vi "TrajectoryParam_calcStuffRev.vi"(6 "TRAJECTORY_CONFIG":T1 {"End Velocity" format="%20.4f"; "StartVelocity" format="%20.4f"; "Max Acceleration" format="%20.4f"; "MaxVelocity" format="%20.4f"}, 7 "Reversed":bool, 9 "successorCONSTRAINED_STATEin":T2={"POSEwCURVATURE"={"CURVATURE"=0.0, "POSE"={"TRANSLATION"={"X"=0.0, "Y"=0.0}, "ROTATION"={"VALUE"=0.0, "COS"=1.0, "SIN"=0.0}}}, "Distance"=0.0, "minAccel"=0.0, "maxAccel"=0.0, "maxVelocity"=0.0} {"POSEwCURVATURE"."POSE"."ROTATION"."SIN" format="%13.4f"; "POSEwCURVATURE"."POSE"."ROTATION"."COS" format="%13.4f"; "POSEwCURVATURE"."POSE"."ROTATION"."VALUE" format="%13.4f"; "POSEwCURVATURE"."POSE"."TRANSLATION"."Y" format="%14.3f"; "POSEwCURVATURE"."POSE"."TRANSLATION"."X" format="%14.3f"}, 11 "thisCONSTRAINED_STATEin":T2={"POSEwCURVATURE"={"CURVATURE"=0.0, "POSE"={"TRANSLATION"={"X"=0.0, "Y"=0.0}, "ROTATION"={"VALUE"=0.0, "COS"=1.0, "SIN"=0.0}}}, "Distance"=0.0, "minAccel"=0.0, "maxAccel"=0.0, "maxVelocity"=0.0} {"POSEwCURVATURE"."POSE"."ROTATION"."SIN" format="%13.4f"; "POSEwCURVATURE"."POSE"."ROTATION"."COS" format="%13.4f"; "POSEwCURVATURE"."POSE"."ROTATION"."VALUE" format="%13.4f"; "POSEwCURVATURE"."POSE"."TRANSLATION"."Y" format="%14.3f"; "POSEwCURVATURE"."POSE"."TRANSLATION"."X" format="%14.3f"}) -> (0 "error out":errorcluster, 1 "successorCONSTRAINED_STATEout":T2={"POSEwCURVATURE"={"CURVATURE"=0.0, "POSE"={"TRANSLATION"={"X"=0.0, "Y"=0.0}, "ROTATION"={"VALUE"=0.0, "COS"=1.0, "SIN"=0.0}}}, "Distance"=0.0, "minAccel"=0.0, "maxAccel"=0.0, "maxVelocity"=0.0} {"POSEwCURVATURE"."POSE"."ROTATION"."SIN" format="%13.4f"; "POSEwCURVATURE"."POSE"."ROTATION"."COS" format="%13.4f"; "POSEwCURVATURE"."POSE"."ROTATION"."VALUE" format="%13.4f"; "POSEwCURVATURE"."POSE"."TRANSLATION"."Y" format="%14.3f"; "POSEwCURVATURE"."POSE"."TRANSLATION"."X" format="%14.3f"}, 3 "thisCONSTRAINED_STATEout":T2={"POSEwCURVATURE"={"CURVATURE"=0.0, "POSE"={"TRANSLATION"={"X"=0.0, "Y"=0.0}, "ROTATION"={"VALUE"=0.0, "COS"=1.0, "SIN"=0.0}}}, "Distance"=0.0, "minAccel"=0.0, "maxAccel"=0.0, "maxVelocity"=0.0} {"POSEwCURVATURE"."POSE"."ROTATION"."SIN" format="%13.4f"; "POSEwCURVATURE"."POSE"."ROTATION"."COS" format="%13.4f"; "POSEwCURVATURE"."POSE"."ROTATION"."VALUE" format="%13.4f"; "POSEwCURVATURE"."POSE"."TRANSLATION"."Y" format="%14.3f"; "POSEwCURVATURE"."POSE"."TRANSLATION"."X" format="%14.3f"})   [LabVIEW 2019, in "Trajectory_Library.lvlib"]
doc: "Internal routine called by TrajectoryParam_timeParam.VI"
uses:
  Trajectory_Library.lvlib
  CONSTRAINED_STATE.ctl
  POSEwCURVATURE.ctl
  POSE2D.ctl
  TRANSLATION2D.ctl
  ROTATION2D.ctl
  TRAJ_CONFIG.ctl
panel:
  # "All units\nare SI"
  # "All units\nare SI"
  # "All units\nare SI"
  # "All units\nare SI"
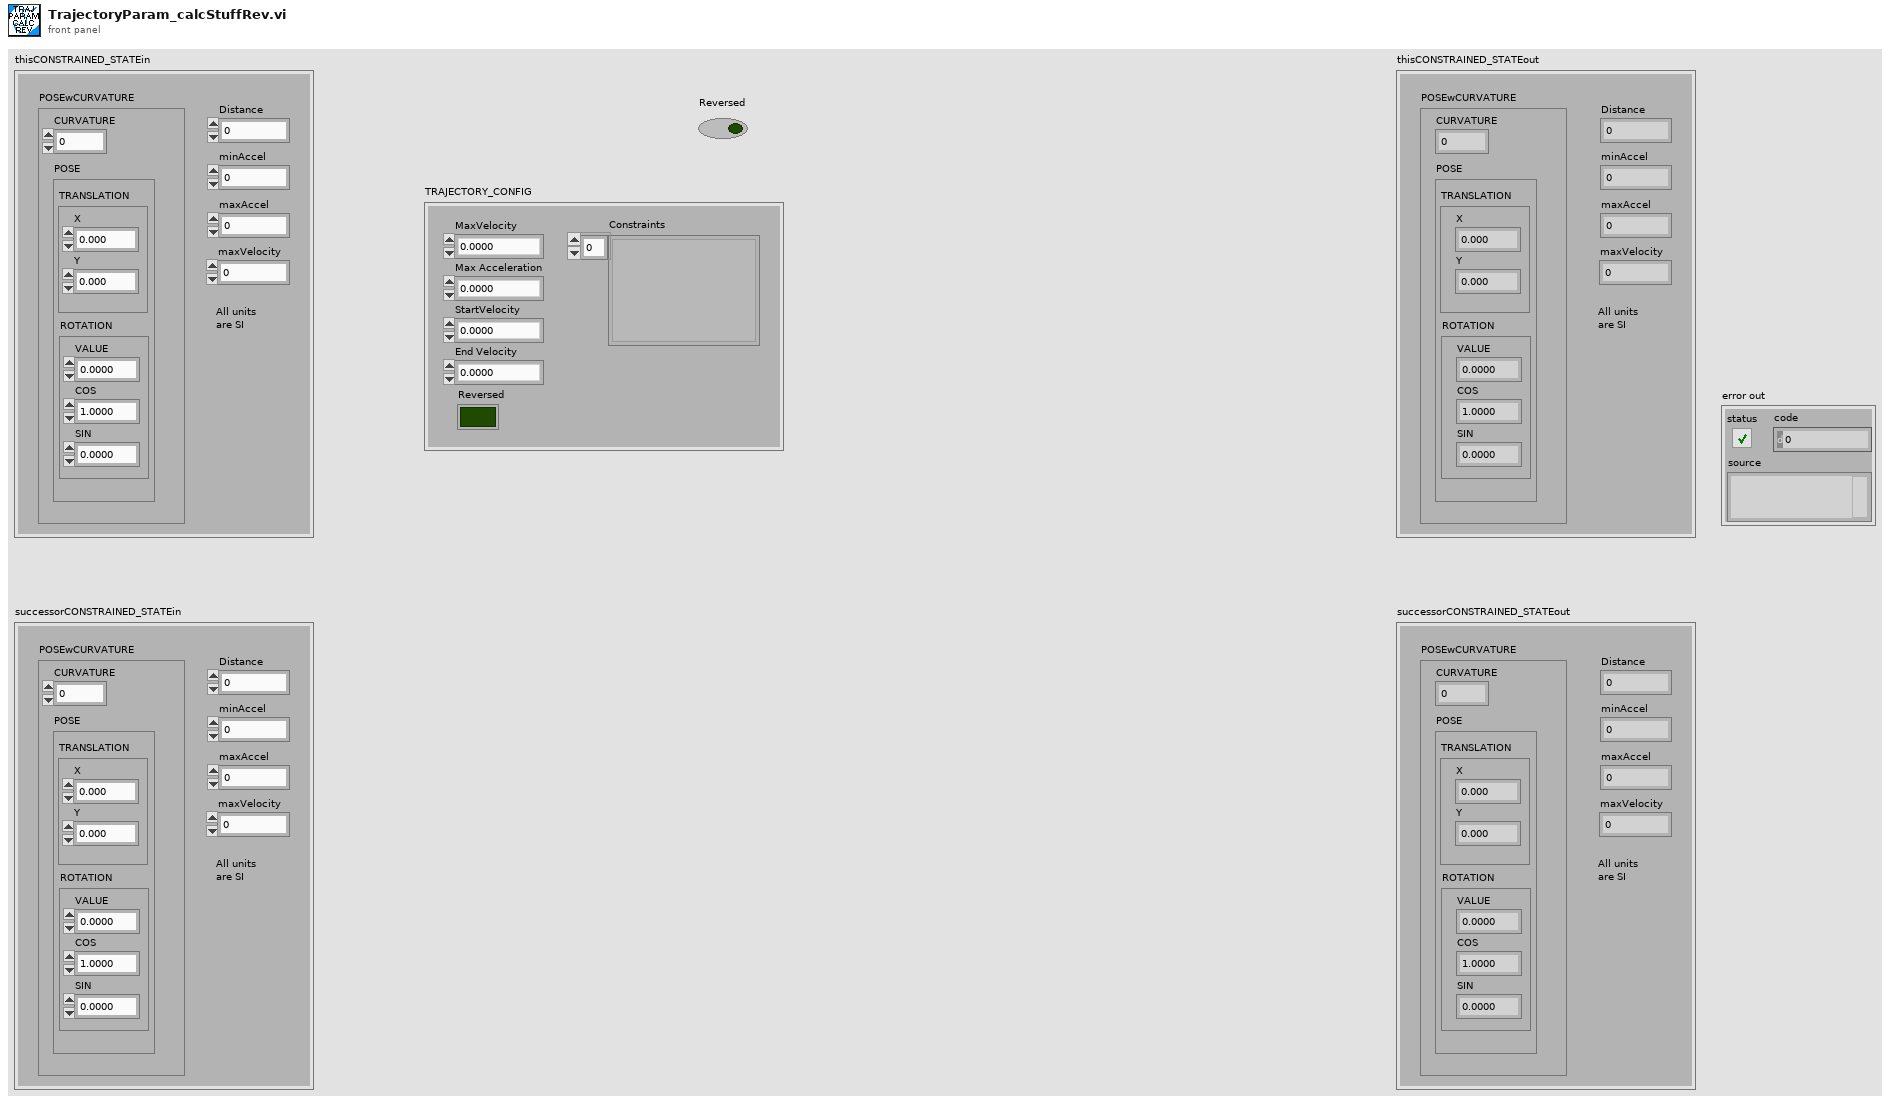
[diagram p1: front panel]
types:
  T1 = typedef "Trajectory_Library.lvlib/TRAJ_CONFIG.ctl" = cluster{"MaxVelocity":dbl, "Max Acceleration":dbl, "StartVelocity":dbl, "End Velocity":dbl, "Reversed":bool, "Constraints":variant[]}
  T2 = typedef "Trajectory_Library.lvlib/CONSTRAINED_STATE.ctl" = cluster{"POSEwCURVATURE":T3, "Distance":dbl, "minAccel":dbl, "maxAccel":dbl, "maxVelocity":dbl}
  T3 = typedef "Trajectory_Library.lvlib/POSEwCURVATURE.ctl" = cluster{"CURVATURE":dbl, "POSE":T4}
  T4 = typedef "Trajectory_Library.lvlib/POSE2D.ctl" = cluster{"TRANSLATION":T5, "ROTATION":T6}
  T5 = typedef "Trajectory_Library.lvlib/TRANSLATION2D.ctl" = cluster{"X":dbl, "Y":dbl}
  T6 = typedef "Trajectory_Library.lvlib/ROTATION2D.ctl" = cluster{"VALUE":dbl, "COS":dbl, "SIN":dbl}
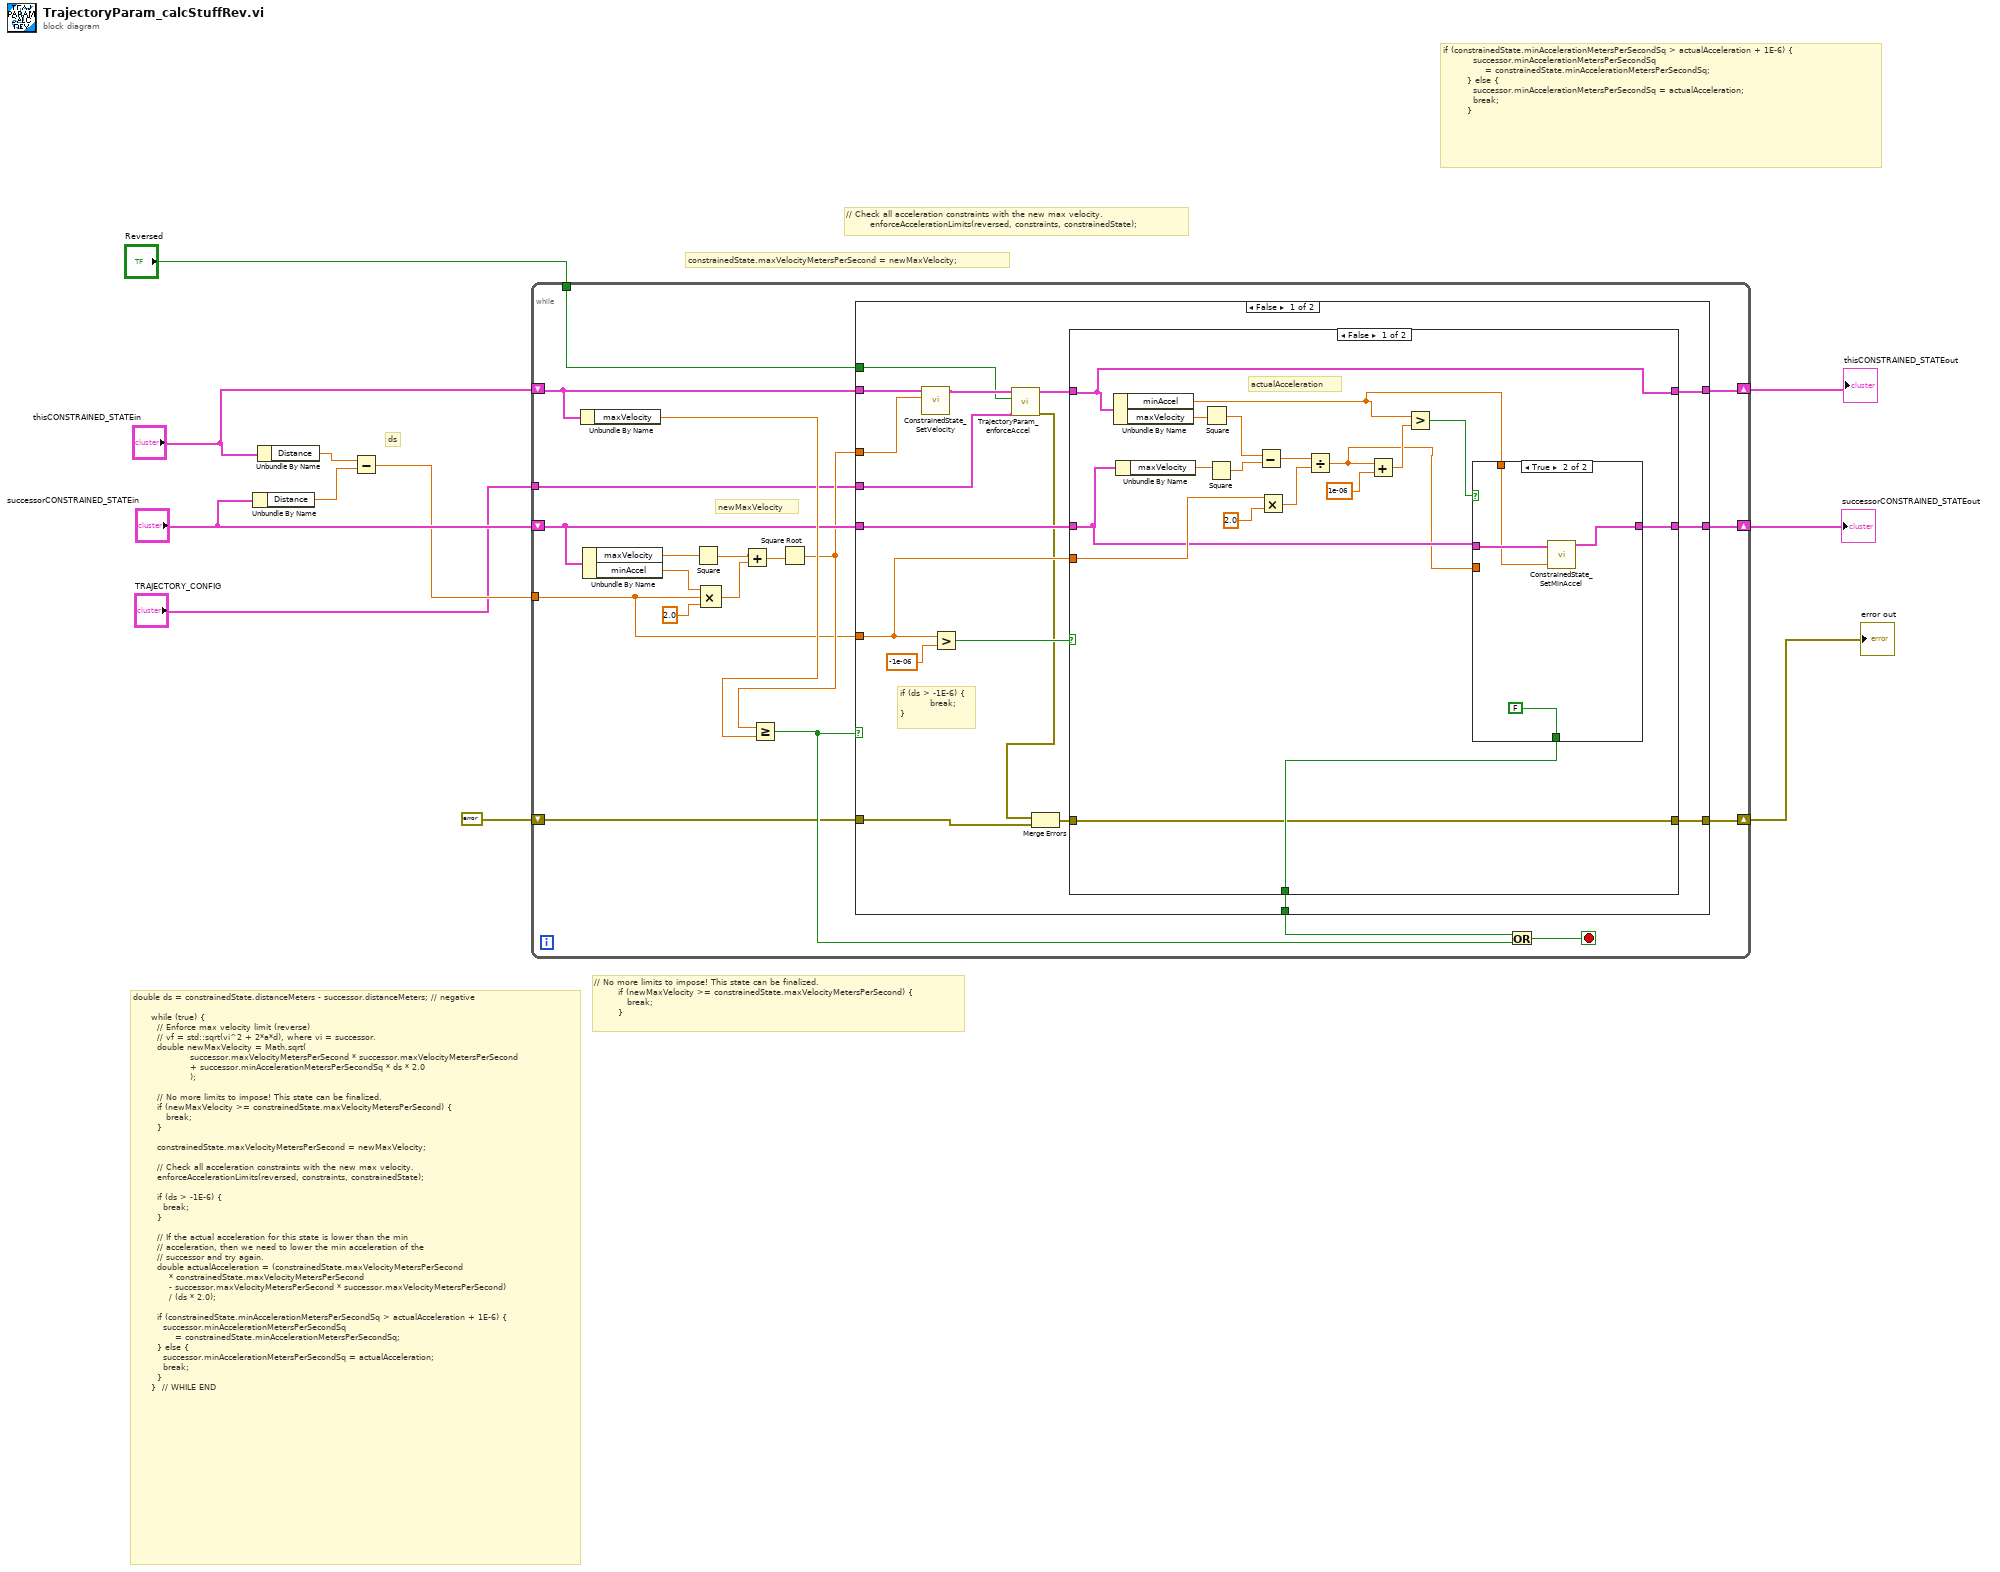
[diagram p0: block diagram]
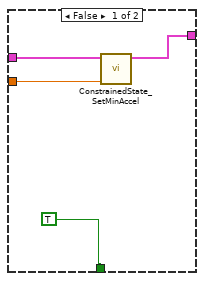
[diagram p2: hidden frame]
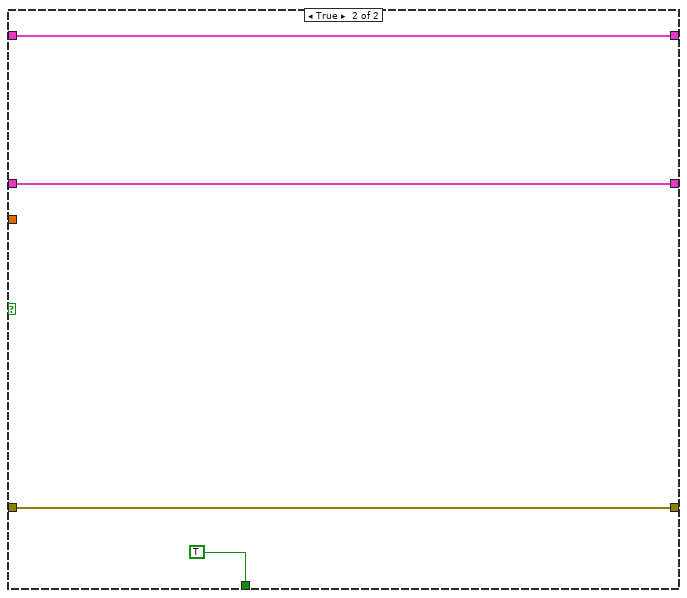
[diagram p3: hidden frame]
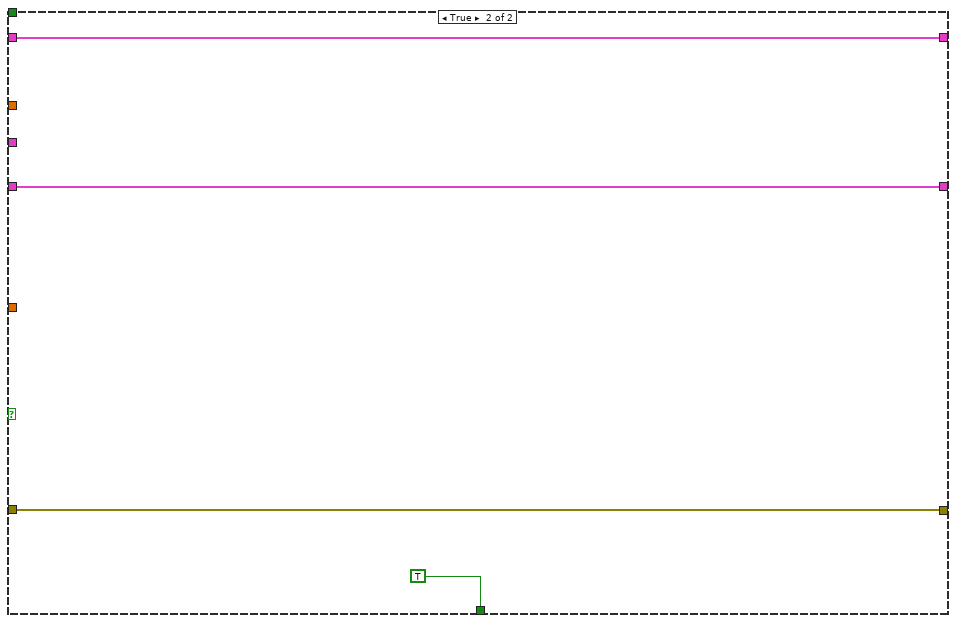
[diagram p4: hidden frame]
diagram:
  # "if (constrainedState.minAccelerationMetersPerSecondSq > actualAcceleration + 1E-6) {\n          successor.minAccelerationMetersPerSecondSq\n              = constrainedState.minAccelerationMetersPerSecondSq;\n        } else {\n          successor.minAccelerationMetersPerSecondSq = actualAcceleration;\n          break;\n        }"
  # "// Check all acceleration constraints with the new max velocity.\n        enforceAccelerationLimits(reversed, constraints, constrainedState);"
  # "constrainedState.maxVelocityMetersPerSecond = newMaxVelocity;"
  # "// No more limits to impose! This state can be finalized.\n        if (newMaxVelocity >= constrainedState.maxVelocityMetersPerSecond) {\n           break;\n        }"
  # "ds"
  # "double ds = constrainedState.distanceMeters - successor.distanceMeters; // negative\n\n      while (true) {\n        // Enforce max velocity limit (reverse)\n        // vf = std::sqrt(vi^2 + 2*a*d), where vi = successor.\n        double newMaxVelocity = Math.sqrt(\n                   successor.maxVelocityMetersPerSecond * successor.maxVelocityMetersPerSecond\n                   + successor.minAccelerationMetersPerSecondSq * ds * 2.0\n                   );\n\n        // No more limits to impose! This state can be finalized.\n        if (newMaxVelocity >= constrainedState.maxVelocityMetersPerSecond) {\n           break;\n        }\n\n        constrainedState.maxVelocityMetersPerSecond = newMaxVelocity;\n\n        // Check all acceleration constraints with the new max velocity.\n        enforceAccelerationLimits(reversed, constraints, constrainedState);\n\n        if (ds > -1E-6) {\n          break;\n        }\n\n        // If the actual acceleration for this state is lower than the min\n        // acceleration, then we need to lower the min acceleration of the\n        // successor and try again.\n        double actualAcceleration = (constrainedState.maxVelocityMetersPerSecond\n            * constrainedState.maxVelocityMetersPerSecond\n            - successor.maxVelocityMetersPerSecond * successor.maxVelocityMetersPerSecond)\n            / (ds * 2.0);\n\n        if (constrainedState.minAccelerationMetersPerSecondSq > actualAcceleration + 1E-6) {\n          successor.minAccelerationMetersPerSecondSq\n              = constrainedState.minAccelerationMetersPerSecondSq;\n        } else {\n          successor.minAccelerationMetersPerSecondSq = actualAcceleration;\n          break;\n        }\n      }  // WHILE END"
  n1 = Unbundle By Name("successorCONSTRAINED_STATEin") -> ("Distance"=w10:dbl)
  n2 = Unbundle By Name("thisCONSTRAINED_STATEin") -> ("Distance"=w11:dbl)
  n3 = Subtract(x=w11, y=w10) -> (x-y=w7:dbl)
  n4 = while {
    shift-right: [w19] -> w4
    shift-left: "successorCONSTRAINED_STATEin" -> [w22]
    shift-right: [w20] -> w5
    shift-left: "thisCONSTRAINED_STATEin" -> [w21]
    tunnel: w7 -> [w16]
    tunnel: "Reversed" -> [w17]
    shift-right: [w13] -> w2
    shift-left: errorcluster {"status"=FALSE, "code"=0, "source"=""} ("error out") -> [w14]
    tunnel: "TRAJECTORY_CONFIG" -> [w12]
    stop <- w25 stop-if-true
    # "newMaxVelocity"
    n5 = Unbundle By Name(w21) -> ("maxVelocity"=w24:dbl)
    n6 = Unbundle By Name(w22) -> ("maxVelocity"=w31:dbl, "minAccel"=w30:dbl)
    n7 = Square(x=w31) -> (x^2=w28:dbl)
    n8 = Compound Arithmetic op=MULTIPLY(w30, w16, 2.0 ("value")) -> (w27:dbl)
    n9 = Add(x=w28, y=w27) -> (x+y=w26:dbl)
    n10 = Square Root(x=w26) -> (sqrt(x)=w18:dbl)
    n11 = Greater Or Equal?(x=w18, y=w24) -> (x >= y?=w23:bool)
    n12 = case shown="False" w23 {
      tunnel: w22 -> [w43 w81]
      tunnel: w21 -> [w48 w82]
      tunnel: [w41 w82] -> w20
      tunnel: [w40 w81] -> w19
      tunnel: w18 -> [w47 _]
      tunnel: w17 -> [w32 _]
      tunnel: w16 -> [w39 _]
      tunnel: [w44 TRUE] -> w15
      tunnel: w14 -> [w38 w79]
      tunnel: [w35 w79] -> w13
      tunnel: w12 -> [w34 _]
      frame False {
        # "if (ds > -1E-6) {\n          break;\n}"
        n13 = call "ConstrainedState_SetVelocity.vi"("maxVelocity"=w47, "inCONSTRAINED_STATE"=w48) -> ("outCONSTRAINED_STATE"=w33:T2)  [unwired: 9 in]
        n14 = Greater?(x=w39, y=-1e-06) -> (0:w45:bool)
        n15 = call "TrajectoryParam_enforceAccel.vi"("TRAJECTORY_CONFIG"=w34, "Reversed"=w32, "inCONSTRAINED_STATE"=w33) -> ("error out"=w37:errorcluster, "outCONSTRAINED_STATE"=w42:T2)  [unwired: 7 in]
        n16 = Merge Errors(w37, w38) -> (w36:errorcluster)
        n17 = case shown="False" w45 {
          tunnel: [w51 TRUE] -> w44
          tunnel: w43 -> [w54 w76]
          tunnel: w42 -> [w56 w77]
          tunnel: [w56 w77] -> w41
          tunnel: [w53 w76] -> w40
          tunnel: w39 -> [w62 _]
          tunnel: w36 -> [w49 w75]
          tunnel: [w49 w75] -> w35
          frame False {
            # "actualAcceleration"
            n18 = Unbundle By Name(w56) -> ("minAccel"=w52:dbl, "maxVelocity"=w66:dbl)
            n19 = Unbundle By Name(w54) -> ("maxVelocity"=w65:dbl)
            n20 = Square(x=w66) -> (x^2=w63:dbl)
            n21 = Square(x=w65) -> (x^2=w64:dbl)
            n22 = Subtract(x=w63, y=w64) -> (x-y=w60:dbl)
            n23 = Multiply(x=w62, y=2.0) -> (x*y=w59:dbl)
            n24 = Divide(x=w60, y=w59) -> (x/y=w50:dbl)
            n25 = Add(x=w50, y=1e-06) -> (x+y=w57:dbl)
            n26 = Greater?(x=w52, y=w57) -> (0:w55:bool)
            n27 = case shown="True" w55 {
              tunnel: w54 -> [w70 w74]
              tunnel: [w69 w73] -> w53
              tunnel: w52 -> [_ w72]
              tunnel: [TRUE FALSE] -> w51
              tunnel: w50 -> [w68 _]
              frame False {
                n28 = call "ConstrainedState_SetMinAccel.vi"("minAcceleration"=w68, "inCONSTRAINED_STATE"=w70) -> ("outCONSTRAINED_STATE"=w69:T2)  [unwired: 9 in]
              }
              frame True {
                n29 = call "ConstrainedState_SetMinAccel.vi"("minAcceleration"=w72, "inCONSTRAINED_STATE"=w74) -> ("outCONSTRAINED_STATE"=w73:T2)  [unwired: 9 in]
              }
            }
          }
          frame True {
          }
        }
      }
      frame True {
      }
    }
    n30 = Or(x=w15, y=w23) -> (x .or. y?=w25:bool)
  }
  "error out" <- w2
  "thisCONSTRAINED_STATEout" <- w5
  "successorCONSTRAINED_STATEout" <- w4
